vi "Main UI.vi"(11 "ABD in":refnum<class "ABD.lvclass">) -> ()   [LabVIEW 2021, in "ABD.lvlib" / "ABD.lvclass"]
uses:
  ABD.lvclass
  ABD.lvclass/ABD.ctl
  LVCAM/Msgs/LVCAM Destroy Self/LVCAM Destroy Self Msg/LVCAM Destroy Self Msg.lvclass
  C:/PPLs/LabVIEW-Composed-Actor-Model-LVCAM/LabVIEW-Composed-Actor-Model-LVCAM/LVCAM/LVCAM/Msg/Msg.lvclass
  LVCAM/LVCAM/Self Actor/Self Msg Send.vi
  LVCAM/LVCAM/Self Actor/Self Actor.lvclass
  C:/PPLs/LabVIEW-Composed-Actor-Model-LVCAM/LabVIEW-Composed-Actor-Model-LVCAM/LVCAM/Msgs/LVCAM Destroy Self/LVCAM Destroy Self Msg/LVCAM Destroy Self Msg.lvclass
  C:/PPLs/LabVIEW-Composed-Actor-Model-LVCAM/LabVIEW-Composed-Actor-Model-LVCAM/LVCAM/Msgs/LVCAM Destroy Self/LVCAM Destroy Self/LVCAM Destroy Self.lvclass
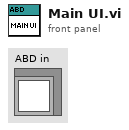
[diagram p1: front panel]
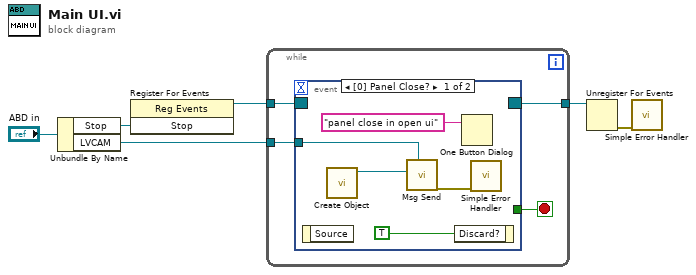
[diagram p0: block diagram]
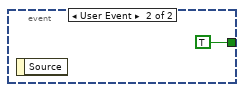
[diagram p2: hidden frame]
diagram:
  n1 = Unbundle By Name("ABD in") -> ("Stop"=w5:refnum<user-event>, "LVCAM"=w2:refnum<class "LVCAM.lvclass">)
  n2 = register-events ("Main Register for Events")(w5) -> (reference out=w4:refnum<event-registration>)  [unwired: 2 in, 1 out]
  n3 = while {
    tunnel: w4 -> [w10]
    tunnel: [w8] -> w6
    tunnel: w2 -> [w7]
    stop <- w9 stop-if-true
    n4 = event "UI Events" shown="[0] Panel Close?" {
      selector: w10 -> [_ _]
      dyn-events: [_ _] -> w8
      timeout: _ -> [_ _]
      tunnel: [_ TRUE] -> w9
      tunnel: w7 -> [w15 _]
      event Panel Close? {
        n5 = event-data() -> ()  [unwired: 1 in, 1 out]
        n6 = call "Create Object.vi"() -> ("LVCAM Destroy Self Msg out"=w11:refnum<class "LVCAM Destroy Self Msg.lvclass">)  [unwired: 11 in]
        n7 = call-poly "Msg Send.vi"("Self Actor"=w15, "Msg"=w11) -> ("error out"=w12:errorcluster)  [unwired: 9 in]
        n8 = event-data("Discard?"=TRUE) -> ()  [unwired: 1 in, 1 out]
        n9 = One Button Dialog(message="panel close in open ui") -> ()  [unwired: 1 in, 1 out]
        n10 = call <vilib>:"Simple Error Handler.vi"("error in (no error)"=w12) -> ()  [unwired: 4 in, 5 out]
      }
      event User Event {
        n11 = event-data() -> ()  [unwired: 1 in, 1 out]
      }
    }
  }
  n12 = Unregister For Events(event registration refnum=w6) -> (error out=w3:errorcluster)  [unwired: 1 in]
  n13 = call <vilib>:"Simple Error Handler.vi"("error in (no error)"=w3) -> ()  [unwired: 4 in, 5 out]
